vi "Recursive_XMLToTree.vi"(9 "Parent Tag":string="*", 10 "Tree Refnum":refnum<vi>, 11 "Node IN":refnum<k20>) -> ()   [LabVIEW 2012]
doc: "SciScan 1.2 160622"
uses:
  <resource>/objmgr/DOMUserDefRef.rc
  <vilib>/xml/NI_XML.lvlib
panel:
  out "error out":errorcluster
  in  "error in (no error)":errorcluster
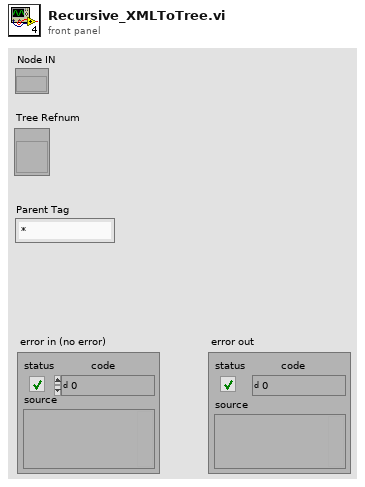
[diagram p1: front panel]
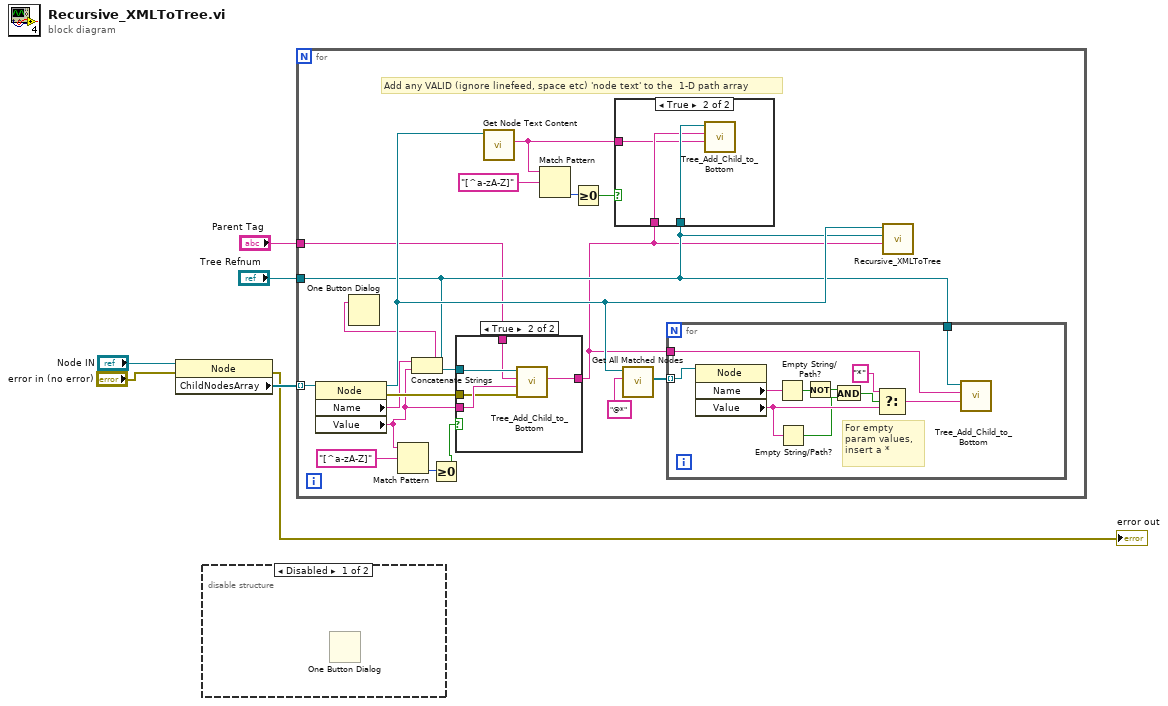
[diagram p0: block diagram]
diagram:
  n1 = property class="Node"(reference="Node IN", error in="error in (no error)") -> (error out=→"error out":errorcluster, "ChildNodesArray"=w5:refnum<k20>[])  [unwired: 1 out]
  n2 = disable-structure shown="Disabled" {
    frame Disabled {
      n3 = One Button Dialog() -> ()  [unwired: 2 in, 1 out]
    }
    frame Enabled {
    }
  }
  n4 = for {
    tunnel: w5 -> [w24] mode=indexing
    tunnel: "Tree Refnum" -> [w15]
    tunnel: "Parent Tag" -> [w14]
    # "Add any VALID (ignore linefeed, space etc) 'node text' to the  1-D path array"
    n5 = property class="Node"(reference=w24) -> (reference out=w16:refnum<k20>, error out=w22:errorcluster, "Name"=w10:string, "Value"=w9:string)  [unwired: 1 in]
    n6 = Match Pattern(string=w9, regular expression="[^a-zA-Z]") -> (offset past match=w13:i32)  [unwired: 1 in, 3 out]
    n7 = Concatenate Strings(w10, w9) -> (w8:string)
    n8 = One Button Dialog(message=w8) -> ()  [unwired: 1 in, 1 out]
    n9 = Greater Or Equal To 0?(x=w13) -> (x >= 0?=w11:bool)
    n10 = case shown="True" w11 {
      tunnel: w15 -> [_ w33]
      tunnel: w14 -> [w28 w32]
      tunnel: w9 -> [_ w31]
      tunnel: w22 -> [_ w30]
      tunnel: [w28 w29] -> w7
      frame False {
      }
      frame True {
        n11 = call "Tree_Add_Child_to_Bottom.vi"("error in (no error)"=w30, "Child String (to add)"=w31, "Parent Tag"=w32, "Tree Refnum IN"=w33) -> ("Newly added Child Tag"=w29:string)  [unwired: 5 in, 2 out]
      }
    }
    n12 = call <vilib>:"Get Node Text Content.vi"("node in"=w16) -> ("node text"=w19:string)  [unwired: 8 in, 2 out]
    n13 = Match Pattern(string=w19, regular expression="[^a-zA-Z]") -> (offset past match=w18:i32)  [unwired: 1 in, 3 out]
    n14 = Greater Or Equal To 0?(x=w18) -> (x >= 0?=w17:bool)
    n15 = case shown="True" w17 {
      tunnel: w19 -> [_ w25]
      tunnel: w15 -> [_ w27]
      tunnel: w7 -> [_ w26]
      frame False {
      }
      frame True {
        n16 = call "Tree_Add_Child_to_Bottom.vi"("Child String (to add)"=w25, "Parent Tag"=w26, "Tree Refnum IN"=w27) -> ()  [unwired: 6 in, 3 out]
      }
    }
    n17 = call <vilib>:"Get All Matched Nodes.vi"("XPath expression"="@*", "node in"=w16) -> ("node result array"=w21:refnum<k20>[])  [unwired: 7 in, 2 out]
    n18 = for {
      tunnel: w21 -> [w37] mode=indexing
      tunnel: w7 -> [w34]
      tunnel: w15 -> [w35]
      # "For empty param values, insert a *"
      n19 = property class="Node"(reference=w37) -> ("Name"=w38:string, "Value"=w43:string)  [unwired: 1 in, 2 out]
      n20 = Empty String/Path?(string/path=w38) -> (empty?=w39:bool)
      n21 = Empty String/Path?(string/path=w43) -> (empty?=w41:bool)
      n22 = Not(x=w39) -> (.not. x?=w40:bool)
      n23 = And(x=w40, y=w41) -> (x .and. y?=w42:bool)
      n24 = Select(t="*", s=w42, f=w43) -> (s? t:f=w36:string)
      n25 = call "Tree_Add_Child_to_Bottom.vi"("Child String (to add)"=w36, "Parent Tag"=w34, "Tree Refnum IN"=w35) -> ()  [unwired: 6 in, 3 out]
    }
    n26 = call "Recursive_XMLToTree.vi"("Parent Tag"=w7, "Tree Refnum"=w15, "Node IN"=w16) -> ()  [unwired: 9 in]
  }
